vi "send.vi"(7 "flags":i32, 8 "error in":errorcluster, 10 "data":string, 11 "socket":i32) -> (0 "error out":errorcluster)   [LabVIEW 2013, in "lvnano.lvlib"]
doc: "NN_EXPORT int nn_send (int s, const void *buf, size_t len, int flags);"
uses:
  lvnano.lvlib
  get last error code.vi
  get error string from code.vi
  <vilib>/Utility/error.llb/Error Cluster From Error Code.vi
  lvnanomsg.dll
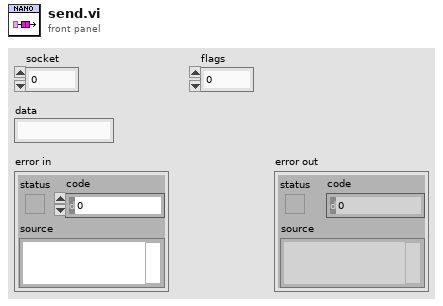
[diagram p1: front panel]
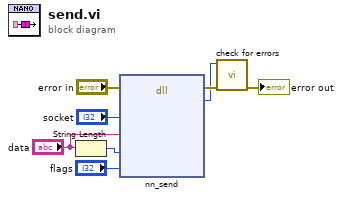
[diagram p0: block diagram]
diagram:
  n1 = String Length(string="data") -> (length=w3:i32)
  n2 = dll-call lib="C:/Users/Daniel/Documents/nanomsg/lvnano/lvnanomsg.*" fn="nn_send"(error in="error in", "socket"="socket", "string"="data", "length"=w3, "flags"="flags") -> (error out=w5:errorcluster, "send count"=w1:i32)  [unwired: 6 in, 1 out]
  n3 = call "check for errors.vi"("error in"=w5, "function return"=w1) -> ("error out"=→"error out":errorcluster)  [unwired: 9 in]
